vi "SOUR_POW_LEV_IMM.vi"(0 "VISA IN":refnum<visa-resource-name>, 3 "Power Level":dbl, 5 "error in":errorcluster, 7 "Channel":i32, 9 "Port number":i32, 11 "Source":string) -> (14 "VISA Out":refnum<visa-resource-name>, 19 "error out":errorcluster)   [LabVIEW 2018, in "PNA-X.lvlib"]
doc: "SOURce<cnum>:POWer<port>[:LEVel][:IMMediate] \n[:AMPLitude] <num>, [src] \n(Read-Write) Sets the RF power output level. \nParameters \n<cnum> Any existing channel number. If unspecified, value is set to 1 \n<port> Port number of the PNA. If unspecified, value is set to 1. To make settings for \nports that are not simple numbers, use the [src] argument. \n<num> Source power in dBm. \nNote: The range of settable power values depends on the PNA model and if \nsource attenuators are installed. To determine the range of values, perform a \nquery using MAX, then MIN, as an argument. (SOUR:POW:ATT:AUTO must \nbe set to ON) Example: SOURce:POWer? Max \nActual achievable leveled power depends on frequency. \n[src] String. (NOT case sensitive). Source port. Optional. Use SOUR:CAT? to \nreturn a list of valid port names. \nWhile this argument can be used to make settings for ALL ports, it is designed \nto access ports that are not simple numbers, such as \"Port 1 Src2\". Otherwise, \nthe <port> argument performs the same function. If both arguments are \nspecified, [src] takes priority.\n1829\n\nExamples SOUR:POW1 5DB \nsource2:power:level:immediate:amplitude maximum \nsour:pow 5, \"Port 1 Src2\" \nQuery Syntax SOURce<cnum>:POWer[:LEVel][:IMMediate][:AMPLitude]? [src] \nReturn Type Numeric \nDefault 0 dBm"
uses:
  PNA-X.lvlib
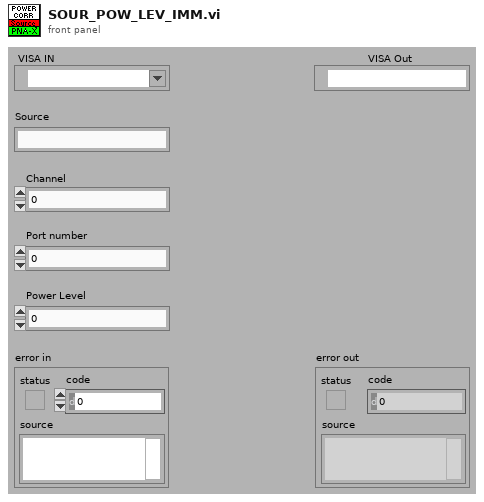
[diagram p1: front panel]
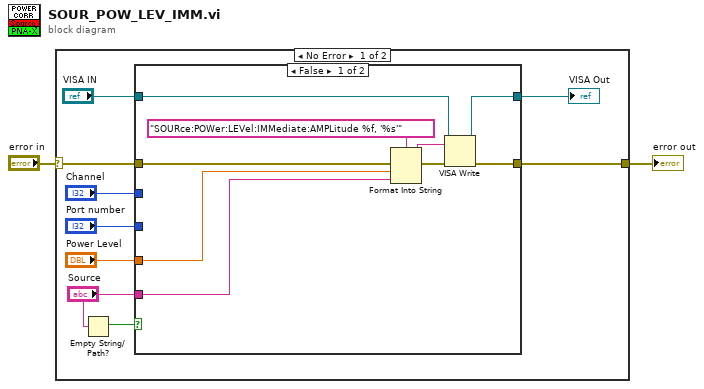
[diagram p0: block diagram]
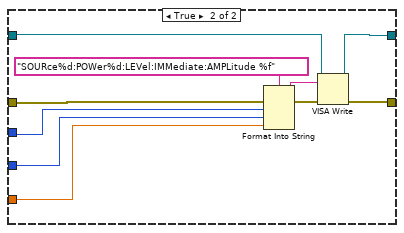
[diagram p2: hidden frame]
diagram:
  n1 = case shown="No Error" "error in" {
    selector: "error in" -> [w11 w31]
    tunnel: [w9 w31] -> w1
    frame No Error {
      n2 = Empty String/Path?(string/path="Source") -> (empty?=w4:bool)
      n3 = case shown="False" w4 {
        tunnel: w11 -> [w20 w27]
        tunnel: "VISA IN" -> [w17 w24]
        tunnel: [w15 w26] -> w9
        tunnel: [w14 w25] -> w8
        tunnel: "Channel" -> [_ w23]
        tunnel: "Port number" -> [_ w22]
        tunnel: "Power Level" -> [w13 w21]
        tunnel: "Source" -> [w12 _]
        frame False {
          n4 = Format Into String(format string="SOURce:POWer:LEVel:IMMediate:AMPLitude %f, '%s'" ("Cmdline"), error in=w20, w13, w12) -> (resulting string=w18:string, error out=w19:errorcluster)  [unwired: 1 in]
          n5 = VISA Write(VISA resource name=w17, write buffer=w18, error in (no error)=w19) -> (VISA resource name out=w14:refnum<visa-resource-name>, error out=w15:errorcluster)  [unwired: 1 out]
        }
        frame True {
          n6 = Format Into String(format string="SOURce%d:POWer%d:LEVel:IMMediate:AMPLitude %f" ("Cmdline"), error in=w27, w23, w22, w21) -> (resulting string=w29:string, error out=w30:errorcluster)  [unwired: 1 in]
          n7 = VISA Write(VISA resource name=w24, write buffer=w29, error in (no error)=w30) -> (VISA resource name out=w25:refnum<visa-resource-name>, error out=w26:errorcluster)  [unwired: 1 out]
        }
      }
      "VISA Out" <- w8
    }
    frame Error {
    }
  }
  "error out" <- w1
